vi "getNewOutCountFile.vi"(10 "Lotno":string) -> (2 "New File":string)   [LabVIEW 2012]
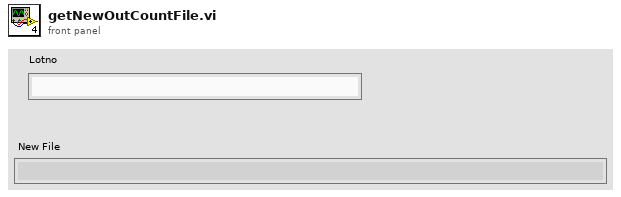
[diagram p1: front panel]
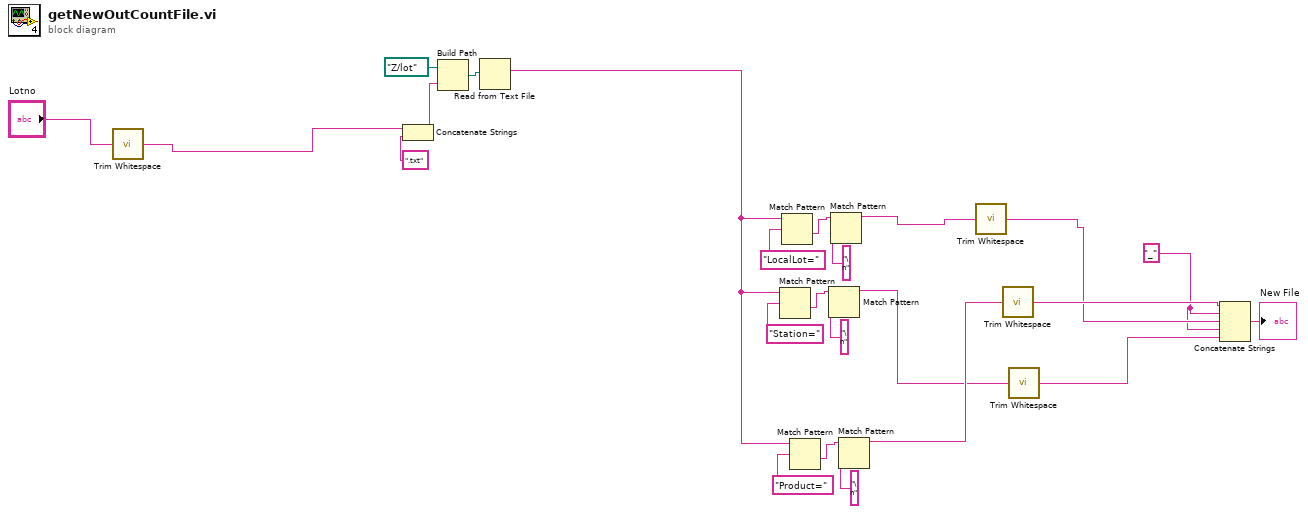
[diagram p0: block diagram]
diagram:
  w7 = "_" ("string")
  n1 = call <vilib>:"Trim Whitespace.vi"("string"="Lotno") -> ("trimmed string"=w2:string)  [unwired: 1 in]
  n2 = Concatenate Strings(w2, ".txt" ("string")) -> (w24:string)
  n3 = Build Path(base path=path "Z:/lot", name or relative path=w24) -> (appended path=w22:path)
  n4 = Read from Text File(file (use dialog)=w22) -> (text=w12:string)  [unwired: 3 in, 3 out]
  n5 = Match Pattern(string=w12, regular expression="Station=") -> (after substring=w17:string)  [unwired: 1 in, 3 out]
  n6 = Match Pattern(string=w12, regular expression="LocalLot=") -> (after substring=w20:string)  [unwired: 1 in, 3 out]
  n7 = Match Pattern(string=w12, regular expression="Product=") -> (after substring=w14:string)  [unwired: 1 in, 3 out]
  n8 = Match Pattern(string=w17, regular expression="\n") -> (before substring=w6:string)  [unwired: 1 in, 3 out]
  n9 = Match Pattern(string=w20, regular expression="\n") -> (before substring=w9:string)  [unwired: 1 in, 3 out]
  n10 = Match Pattern(string=w14, regular expression="\n") -> (before substring=w11:string)  [unwired: 1 in, 3 out]
  n11 = call <vilib>:"Trim Whitespace.vi"("string"=w9) -> ("trimmed string"=w8:string)  [unwired: 1 in]
  n12 = call <vilib>:"Trim Whitespace.vi"("string"=w11) -> ("trimmed string"=w10:string)  [unwired: 1 in]
  n13 = call <vilib>:"Trim Whitespace.vi"("string"=w6) -> ("trimmed string"=w5:string)  [unwired: 1 in]
  n14 = Concatenate Strings(w10, w7, w8, w7, w5) -> (→"New File":string)
